vi "m04gis.vi"(11 "EV3 in":T1) -> ()   [LabVIEW 2016]
uses:
  <vilib>/NXT/Subs/LVHSConnector.ctl
  <vilib>/NXT/LegoClasses/BrickReference/BrickReference.lvclass
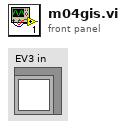
[diagram p1: front panel]
types:
  T1 = typedef "LVHSConnector.ctl" = refnum<class "BrickReference.lvclass">
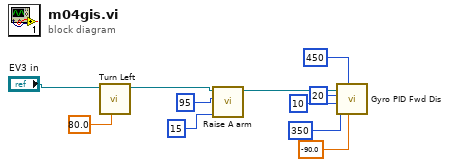
[diagram p0: block diagram]
diagram:
  n1 = call "Turn Left.vi"("Turning angle"=sgl 80.0, "EV3 in"="EV3 in") -> ("EV3 out"=w2:T1)  [unwired: 9 in]
  n2 = call "Raise A arm.vi"("Power"=i8 15, "Rotation"=95, "EV3 in"=w2) -> ("EV3 out"=w1:T1)  [unwired: 8 in]
  n3 = call "Gyro PID Fwd Dis.vi"("Target angle"=sgl -90.0, "Threshold to stop"=450, "Threshold to slow"=350, "Min. speed"=10, "Max. speed"=20, "EV3 in"=w1) -> ()  [unwired: 5 in, 1 out]
